vi "cDAQ DDS Process Status.vi"(8 "error in":errorcluster, 11 "cDAQ dds":T1={"device"="", "channels"=[], "mclk source"="", "mclk [Hz]"=0.0, "fs [Hz]"=0.0, "block [s]"=0.0, "buf [s]"=0.0, "task"="", "cmd queue"=refnum, "proc ref"=refnum, "smpl clock out"="/cDAQ3/PFI0", "export smpl clock"=FALSE, "DC ofs [V]"=[], "timebase source"="", "timebase mode"=enum."Local"} {"channels" min=0 step=1}) -> (0 "error out":errorcluster, 1 "sweep error out":errorcluster, 3 "is running":bool)   [LabVIEW 2013]
uses:
  cDAQ DDS Session.ctl
  cDAQ DDS Setup.ctl
  cDAQ DDS Timebase Mode.ctl
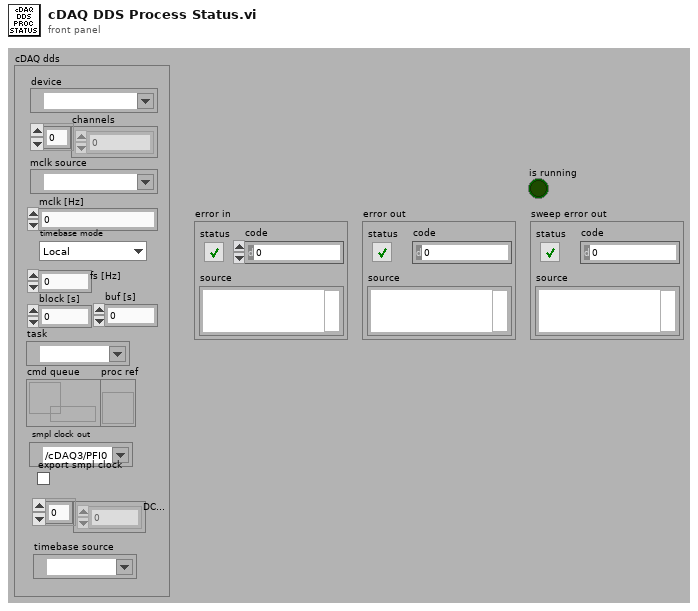
[diagram p1: front panel]
types:
  T1 = typedef "cDAQ DDS Session.ctl" = cluster{"device":tag, "channels":i32[], "mclk source":tag, "mclk [Hz]":dbl, "fs [Hz]":dbl, "block [s]":dbl, "buf [s]":dbl, "task":refnum<k21>, "cmd queue":refnum<queue>, "proc ref":refnum<vi>, "smpl clock out":tag, "export smpl clock":bool, "DC ofs [V]":dbl[], "timebase source":tag, "timebase mode":T2}
  T2 = typedef "cDAQ DDS Timebase Mode.ctl" = enum16{"Local", "Take from ADC (e.g. NI 9238)", "Other source"}
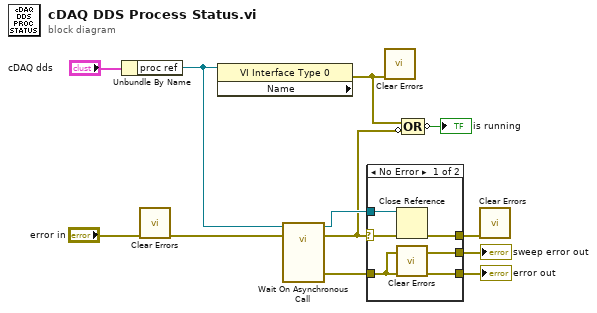
[diagram p0: block diagram]
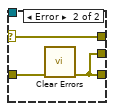
[diagram p2: hidden frame]
diagram:
  n1 = Unbundle By Name("cDAQ dds") -> ("proc ref"=w4:refnum<vi>)
  n2 = call <vilib>:"Clear Errors.vi"("error in (no error)"="error in") -> ("error out"=w7:errorcluster)  [unwired: 6 in]
  n3 = property class="VI Interface Type 0" props=["Name"](reference=w4) -> (error out=w3:errorcluster)  [unwired: 1 in, 2 out]
  n4 = call-by-ref "Wait On Asynchronous Call"(reference=w4, error in=w7) -> (reference out=w10:refnum<vi>, error out=w2:errorcluster, 0:"error out"=w8:errorcluster)  [unwired: 11 in]
  n5 = case shown="No Error" w2 {
    selector: w2 -> [w17 w20]
    tunnel: w10 -> [w16 _]
    tunnel: [w15 w20] -> w9
    tunnel: [w13 w18] -> w12
    tunnel: w8 -> [w14 w19]
    tunnel: [w14 w18] -> w11
    frame No Error {
      n6 = Close Reference(reference=w16, error in (no error)=w17) -> (error out=w15:errorcluster)
      n7 = call <vilib>:"Clear Errors.vi"("error in (no error)"=w14) -> ("error out"=w13:errorcluster)  [unwired: 6 in]
    }
    frame Error {
      n8 = call <vilib>:"Clear Errors.vi"("error in (no error)"=w19) -> ("error out"=w18:errorcluster)  [unwired: 6 in]
    }
  }
  "error out" <- w12
  "sweep error out" <- w11
  n9 = call <vilib>:"Clear Errors.vi"("error in (no error)"=w3) -> ()  [unwired: 6 in, 1 out]
  n10 = Compound Arithmetic op=OR(w3, invert w2) -> (invert →"is running":bool)
  n11 = call <vilib>:"Clear Errors.vi"("error in (no error)"=w9) -> ()  [unwired: 6 in, 1 out]
